vi "quadratic equation.vi"() -> ()   [LabVIEW 2018]
uses:
  RPN/RPN.lvlib
panel:
  out "formula 2":string
  out "formula 1":string
  out "r2":dbl
  out "r1":dbl
  in  "c":i32
  in  "b":i32
  in  "a":i32
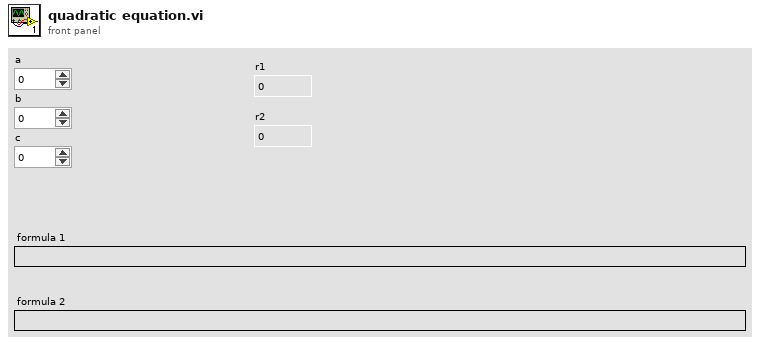
[diagram p1: front panel]
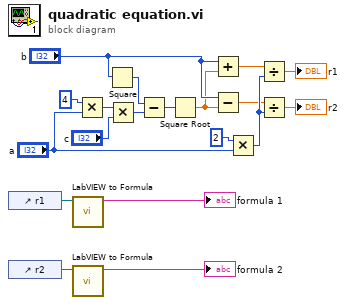
[diagram p0: block diagram]
diagram:
  n1 = control-ref of="r1"() -> (w3:refnum<vi>)
  n2 = control-ref of="r2"() -> (w4:refnum<vi>)
  n3 = call "LabVIEW to Formula.vi"("output ref"=w3) -> ("element"=→"formula 1":string)  [unwired: 10 in]
  n4 = call "LabVIEW to Formula.vi"("output ref"=w4) -> ("element"=→"formula 2":string)  [unwired: 10 in]
  n5 = Multiply(x=u8 4, y="a") -> (x*y=w16:i32)
  n6 = Square(x="b") -> (x^2=w12:i32)
  n7 = Multiply(x=w16, y="c") -> (x*y=w11:i32)
  n8 = Subtract(x=w12, y=w11) -> (x-y=w13:i32)
  n9 = Square Root(x=w13) -> (sqrt(x)=w2:dbl)
  n10 = Add(x="b", y=w2) -> (x+y=w8:dbl)
  n11 = Subtract(x="b", y=w2) -> (x-y=w1:dbl)
  n12 = Multiply(x=u8 2, y="a") -> (x*y=w7:i32)
  n13 = Divide(x=w8, y=w7) -> (x/y=→"r1":dbl)
  n14 = Divide(x=w1, y=w7) -> (x/y=→"r2":dbl)
